vi "Flock_LocalProcess1_Process.vi"(11 "Process":string) -> ()   [LabVIEW 2013, in "FA_Local Process.lvlib"]
uses:
  FA_Local Process.lvlib
  Shared Code/AMC/VI Source/LocalProcessMessaging/Flock_Shared_LocalProcessMessaging.lvlib
  Shared Code/AMC/VI Source/CentralProcessMessaging/Flock_Shared_CentralProcessMessaging.lvlib
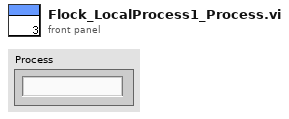
[diagram p1: front panel]
types:
  T1 = typedef "Flock_Shared_Messaging.lvlib/ProcessList.ctl" = string
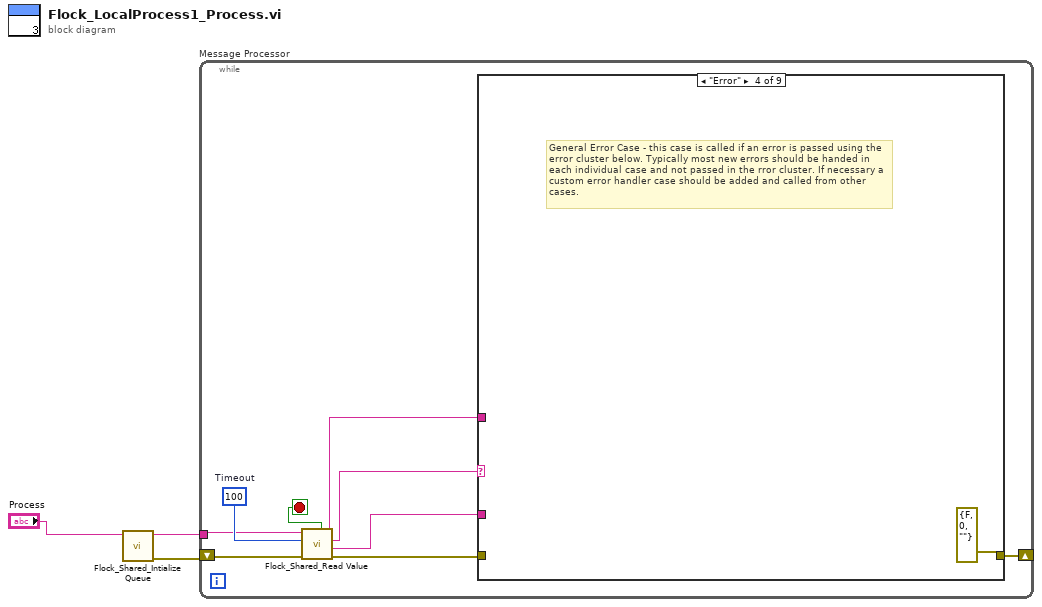
[diagram p0: block diagram]
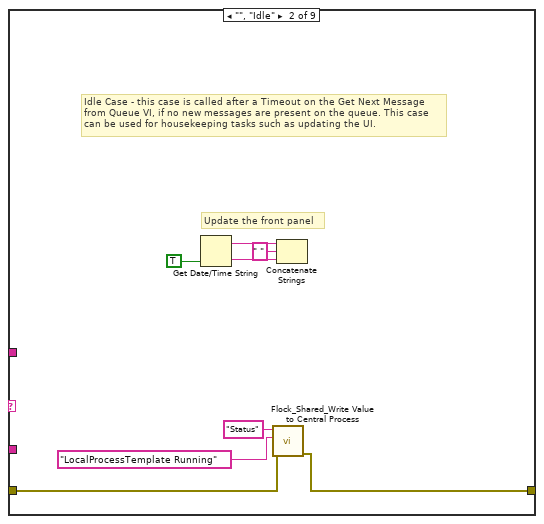
[diagram p3: hidden frame]
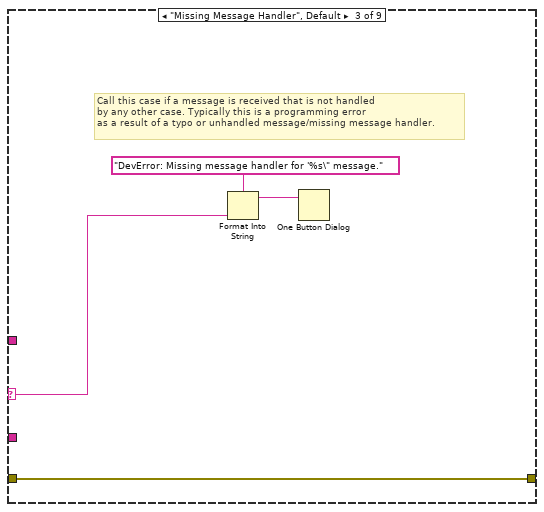
[diagram p4: hidden frame]
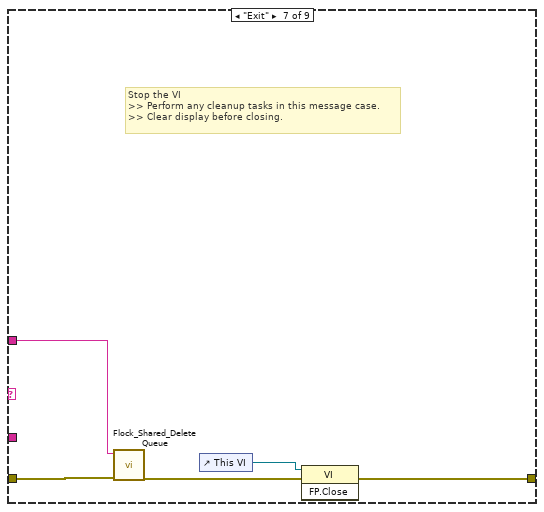
[diagram p7: hidden frame]
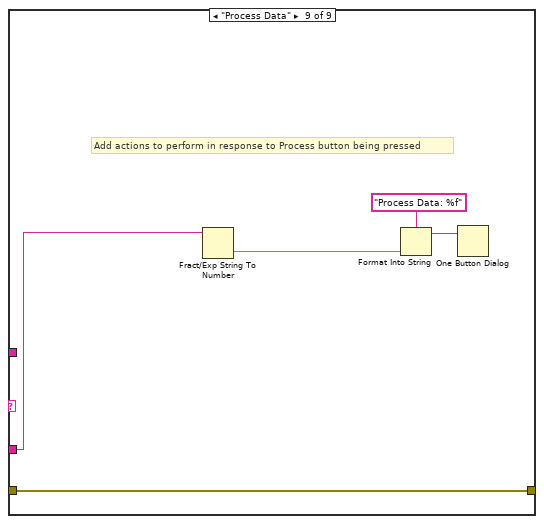
[diagram p9: hidden frame]
diagram:
  n1 = call "Flock_Shared_Intialize Queue.vi"("Enum"="Process") -> ("error out"=w2:errorcluster, "Process Name"=w1:T1)  [unwired: 9 in]
  n2 = while "Message Processor" {
    shift-left: w2 -> [w10]
    shift-right: [w12] -> _
    tunnel: w1 -> [w5]
    stop <- w6 stop-if-true
    w11 = 100  # Timeout
    n3 = call "Flock_Shared_Read Value.vi"("error in (no error)"=w10, "timeout (1ms)"=w11, "Process"=w5) -> ("error out"=w9:errorcluster, "Message Value"=w7:string, "Message Name"=w8:string, "Process"=w4:T1, "Exit Process"=w6:bool)  [unwired: 4 in]
    n4 = case shown="\"Error\"" w8 {
      selector: w8 -> [_ _ w25 _ _ _ _ _ _]
      tunnel: [w13 w14 w22 errorcluster {"status"=FALSE, "code"=0, "source"=""} ("error out") w27 w28 w29 w34 w36] -> w12
      tunnel: w9 -> [w13 w15 w22 _ w27 w28 w33 w34 w36]
      tunnel: w7 -> [_ _ _ _ _ _ _ _ w35]
      tunnel: w4 -> [_ _ _ _ _ _ w32 _ _]
      frame "---------- Framework Operations ----------" {
        # "Dummy case to add a seperator in the Case Structure menu"
      }
      frame "", "Idle" {
        # "Update the front panel"
        # "Idle Case - this case is called after a Timeout on the Get Next Message from Queue VI, if no new messages are present on the queue. This case can be used for housekeeping tasks such as updating the UI."
        n5 = Get Date/Time String(want seconds? (F)=TRUE) -> (date string=w21:string, time string=w20:string)  [unwired: 2 out]
        n6 = call "Flock_Shared_Write Value to Central Process.vi"("error in (no error)"=w15, "Message Value"="LocalProcessTemplate Running", "Message Name"="Status") -> ("error out"=w14:errorcluster)  [unwired: 8 in]
        n7 = Concatenate Strings(w21, " " ("string"), w20) -> ()  [unwired: 1 out]
      }
      frame "Missing Message Handler", Default {
        # "Call this case if a message is received that is not handled \nby any other case. Typically this is a programming error\nas a result of a typo or unhandled message/missing message handler."
        n8 = Format Into String(format string="DevError: Missing message handler for '%s\" message." ("message"), w25) -> (resulting string=w23:string)  [unwired: 2 in, 1 out]
        n9 = One Button Dialog(message=w23) -> ()  [unwired: 2 out]
      }
      frame "Error" {
        # "General Error Case - this case is called if an error is passed using the error cluster below. Typically most new errors should be handed in each individual case and not passed in the rror cluster. If necessary a custom error handler case should be added and called from other cases."
      }
      frame "---------- Generic Operations ----------" {
        # "Dummy case to add a seperator in the Case Structure menu"
      }
      frame "Initialize" {
        # "Initialize the state variables and user interface"
      }
      frame "Exit" {
        # "Stop the VI\n>> Perform any cleanup tasks in this message case.\n>> Clear display before closing."
        n10 = call "Flock_Shared_Delete Queue.vi"("Error In"=w33, "Process Name"=w32) -> ("Error Out"=w30:errorcluster)  [unwired: 9 in]
        n11 = control-ref of="This VI"() -> (w31:refnum<vi>)
        n12 = invoke class="VI" method="FP.Close"(reference=w31, error in=w30) -> (error out=w29:errorcluster)  [unwired: 1 in, 2 out]
      }
      frame "---------- Application Operations ----------" {
        # "Dummy case to add a seperator in the Case Structure menu"
      }
      frame "Process Data" {
        # "Add actions to perform in response to Process button being pressed"
        n13 = Fract/Exp String To Number(string=w35) -> (number=w39:dbl)  [unwired: 4 out]
        n14 = Format Into String(format string="Process Data: %f" ("message"), w39) -> (resulting string=w37:string)  [unwired: 2 in, 1 out]
        n15 = One Button Dialog(message=w37) -> ()  [unwired: 2 out]
      }
    }
  }
